vi "Generate Patch Sequence Images-retd.vi"(4 "Green":path[](array[path]), 5 "Red":path[](array[path]), 6 "Predominant ROI type":T1=enum."Comp. volume", 7 "Imaging Protocol":T2=enum."Live Imaging", 8 "error in (no error)":errorcluster, 9 "Green TIFF handles":i32[](array[numeric]), 10 "Red TIFF handles":i32[](array[numeric]), 11 "TDMS file path & name":path) -> (0 "error out":errorcluster, 2 "Destination fiolder":path)   [LabVIEW 2020]
uses:
  Typedefs/Imaging Protocols enum.ctl
  Typedefs/ROI ID Enum.ctl
  User Interface/Visualisation/Functional Imaging Viewer/SubVIs/Experiment header interface/Typedefs/Save-Load-Save as-Load last enum.ctl
  User Interface/Visualisation/Functional Imaging Viewer/SubVIs/Experiment header interface/Typedefs/Header file type enum.ctl
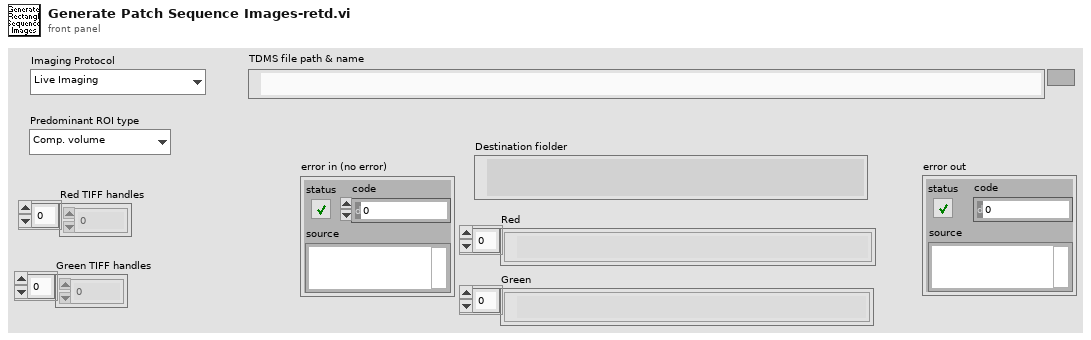
[diagram p1: front panel]
types:
  T1 = typedef "ROI ID Enum.ctl" = enum16{"Point", "MiniScan", "Comp. MiniScan", "Rectangle", "Comp. volume", "Arb. plane point", "None"}
  T2 = typedef "Imaging Protocols enum.ctl" = enum16{"AOL Z-Stack", "Motor Z Stack", "Functional Acquisition", "Single Plane Acquisition", "Volume Acquisition", "Live Imaging", "Live Plane Imaging", "Live Volume Imaging"}
  T3 = typedef "Header file type enum.ctl" = enum16{"All parameters", "Params for funct acq w ROI or mscn", "Params for funct acq w rectangles", "Live imaging header parameters", "AOL Parameters"}
  T4 = typedef "Header file type enum.ctl" = enum16{"All parameters", "Login", "Global Parameters", "Imaging Modes", "Time Series", "Motor Zstack", "AOL Zstack", "Functional Imaging", "Movement Correction", "Calibration Setup", "Statistics", "Biology Information"}
  T5 = typedef "Save-Load-Save as-Load last enum.ctl" = enum16{"Save file", "Save file as", "Load file", "Load last file"}
  T6 = typedef "Header parameters cluster-ALL-retd.ctl" = cluster{"Imaging Protocol":T2, "Number of POI":u16, "Number of Miniscans":u16, "Number of Trials":u16, "Number of Cycles ":u64, "# Averaged Frames":u16, "Laser power (%)":u8, "Pockels":dbl, "Acquisition Length (sec)":dbl, "Fill time (us)":dbl, "POI Dwell time (us)":dbl, "Miniscan Dwell time per pixel (us)":dbl, "PMT 1":dbl, "PMT 2":dbl, "Back Apperture":dbl, "Zoom":dbl, "Frame Size":T7, "Center Frequency":dbl, "Field of View":dbl, "DwellTime (us)":dbl, "Wavelength (nm)":dbl, "AOL Z":dbl, "AOL Mode":T8, "GridXY":dbl, "GridZ":dbl, "TriggerDelay (sec)":dbl, "Number of Pixels in Miniscan":u16, "Experiment folder path":path, "X centre":dbl, "Y centre":dbl, "Angle (degrees)":dbl, "Plane Mode":T9, "Software version":dbl, "Objective":T10, "MotorZ Calibration":u32, "Pockels Calibration":u32, "Threshold":u16[], "Video length (sec)":dbl, "Frame rate (fps)":u8, "Rectangle ROI length (pixels)":u16, "Rectangle ROI height (pixels)":u16}
  T7 = typedef "Frame Size.ctl" = u16
  T8 = typedef "AOL modes.ctl" = enum16{"Raster", "Structural", "Pointing", "Mini Scan", "Alignment"}
  T9 = typedef "Plane Mode.ctl" = u16
  T10 = typedef "Objective selector control enum.ctl" = string
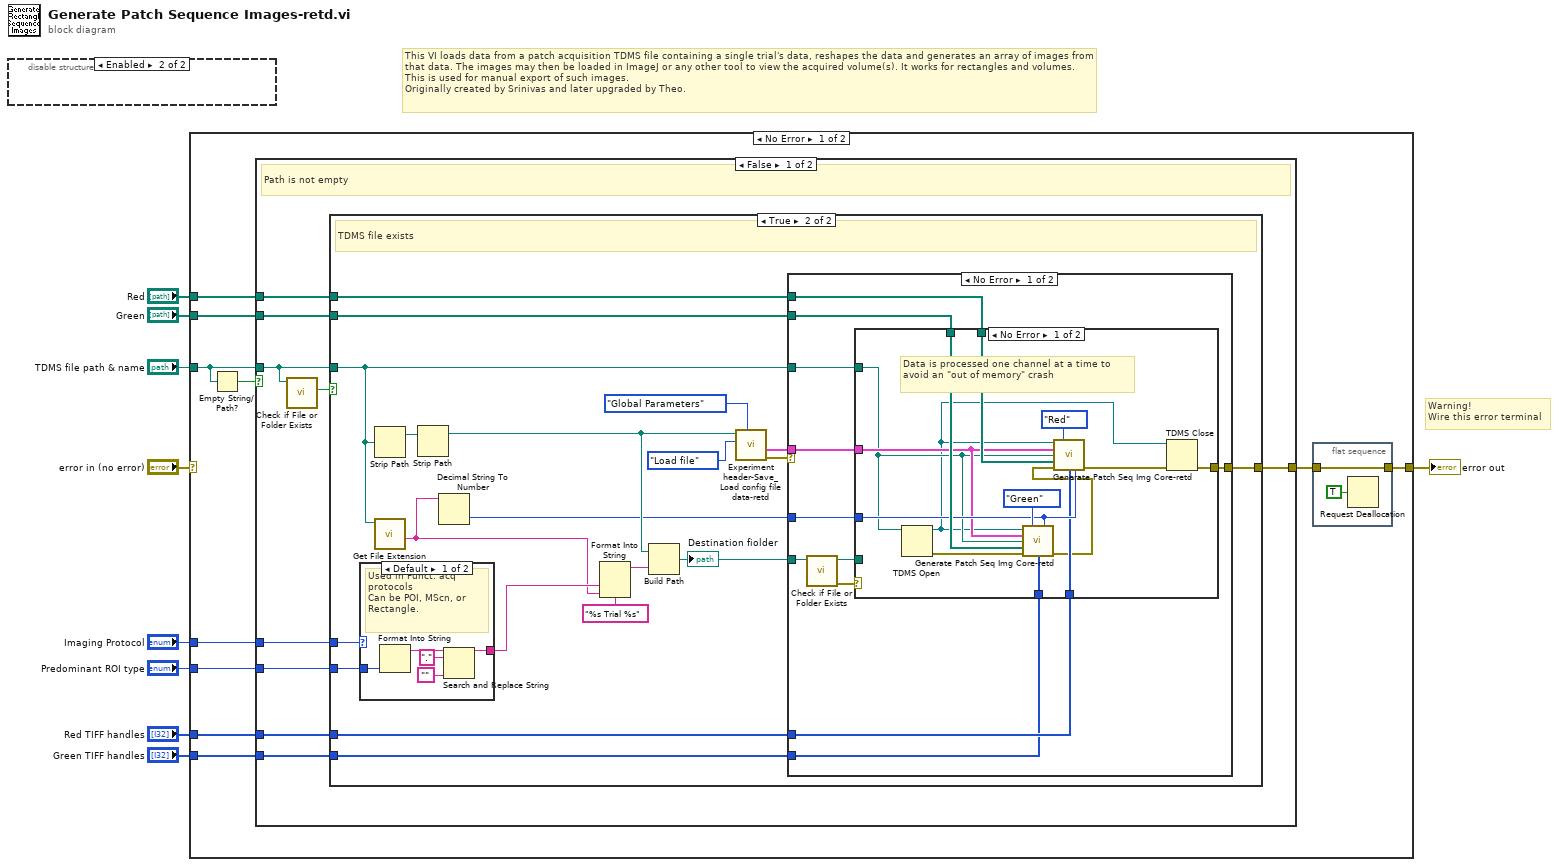
[diagram p0: block diagram]
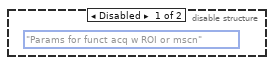
[diagram p2: hidden frame]
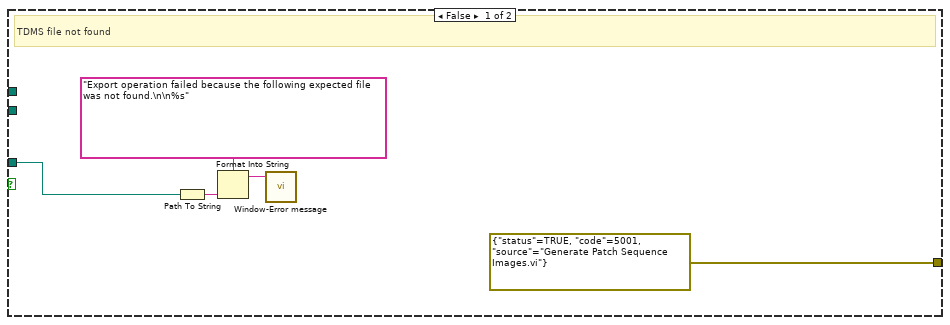
[diagram p3: hidden frame]
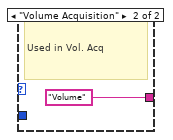
[diagram p6: hidden frame]
diagram:
  # "This VI loads data from a patch acquisition TDMS file containing a single trial's data, reshapes the data and generates an array of images from that data. The images may then be loaded in ImageJ or any other tool to view the acquired volume(s). It works for rectangles and volumes. This is used for manual export of such images.\nOriginally created by Srinivas and later upgraded by Theo."
  # "Warning!\nWire this error terminal"
  n1 = disable-structure shown="Enabled" {
    frame Disabled {
      (unwired) Header_file_type_enum."Params for funct acq w ROI or mscn" ("Header file type")
    }
    frame Enabled {
    }
  }
  n2 = case shown="No Error" "error in (no error)" {
    selector: "error in (no error)" -> [_ w88]
    tunnel: "TDMS file path & name" -> [w18 _]
    tunnel: "Imaging Protocol" -> [w17 _]
    tunnel: "Predominant ROI type" -> [w16 _]
    tunnel: "Green" -> [w14 _]
    tunnel: "Red" -> [w13 _]
    tunnel: "Red TIFF handles" -> [w12 _]
    tunnel: "Green TIFF handles" -> [w11 _]
    tunnel: [w10 w88] -> w2
    frame No Error {
      n3 = Empty String/Path?(string/path=w18) -> (empty?=w19:bool)
      n4 = case shown="False" w19 {
        tunnel: w18 -> [w29 _]
        tunnel: [w28 _] -> w15
        tunnel: w17 -> [w27 _]
        tunnel: w16 -> [w26 _]
        tunnel: w14 -> [w25 _]
        tunnel: w13 -> [w24 _]
        tunnel: w12 -> [w23 _]
        tunnel: w11 -> [w22 _]
        frame False {
          # "Path is not empty"
          n5 = call <vilib>:"Check if File or Folder Exists.vi"("path"=w29) -> ("file or folder exists?"=w30:bool)  [unwired: 8 in, 2 out]
          n6 = case shown="True" w30 {
            tunnel: w29 -> [w34 w55]
            tunnel: [errorcluster {"status"=TRUE, "code"=5001, "source"="Generate Patch Sequence Images.vi"} ("error IO") w53] -> w28
            tunnel: w27 -> [_ w51]
            tunnel: w26 -> [_ w50]
            tunnel: w25 -> [_ w49]
            tunnel: w24 -> [_ w48]
            tunnel: w23 -> [_ w39]
            tunnel: w22 -> [_ w38]
            frame False {
              # "TDMS file not found"
              n7 = Path To String(path=w34) -> (string=w33:string)
              n8 = Format Into String(format string="Export operation failed because the following expected file was not found.\n\n%s", w33) -> (resulting string=w32:string)  [unwired: 2 in, 1 out]
              n9 = call "Window-Error message.vi"("Message"=w32) -> ()  [unwired: 10 in, 1 out]
            }
            frame True {
              # "TDMS file exists"
              n10 = case shown="Default" w51 {
                tunnel: w50 -> [w86 _]
                tunnel: [w82 "Volume" ("result string")] -> w44
                frame Default {
                  # "Used in Funct. acq protocols\nCan be POI, MScn, or Rectangle."
                  n11 = Format Into String(w86) -> (resulting string=w85:string)  [unwired: 3 in, 1 out]
                  n12 = Search and Replace String(input string=w85, search string=".", replace string="" ("replace string (\"\")")) -> (result string=w82:string)  [unwired: 5 in, 3 out]
                }
                frame "Volume Acquisition" {
                  # "Used in Vol. Acq"
                }
              }
              n13 = Strip Path(path=w55) -> (stripped path=w46:path)  [unwired: 1 out]
              n14 = call <vilib>:"Get File Extension.vi"("file"=w55) -> ("filename without extension"=w42:string)  [unwired: 6 in, 4 out]
              n15 = Strip Path(path=w46) -> (stripped path=w54:path)  [unwired: 1 out]
              n16 = Decimal String To Number(string=w42) -> (number=w47:i32)  [unwired: 2 in, 1 out]
              n17 = Format Into String(format string="%s Trial %s", w44, w42) -> (resulting string=w43:string)  [unwired: 2 in, 1 out]
              n18 = Build Path(base path=w54, name or relative path=w43) -> (appended path=w52:path)
              "Destination fiolder" <- w52
              n19 = call "Experiment header-Save_Load config file data-retd.vi"("Header file type"=Header_file_type_enum."Global Parameters", "Function"=Save-Load-Save_as-Load_last_enum."Load file", "Experiment data folder path"=w54) -> ("error out"=w40:errorcluster, "All header parameters out"=w41:T6)  [unwired: 7 in]
              n20 = case shown="No Error" w40 {
                tunnel: w52 -> [w66 _]
                tunnel: w55 -> [w65 _]
                tunnel: w41 -> [w63 _]
                tunnel: [w64 _] -> w53
                tunnel: w49 -> [w62 _]
                tunnel: w48 -> [w61 _]
                tunnel: w47 -> [w60 _]
                tunnel: w39 -> [w57 _]
                tunnel: w38 -> [w56 _]
                frame No Error {
                  n21 = call <vilib>:"Check if File or Folder Exists.vi"("path"=w66) -> ("error out"=w58:errorcluster, "dup path"=w59:path)  [unwired: 8 in, 1 out]
                  n22 = case shown="No Error" w58 {
                    selector: w58 -> [_ w81]
                    tunnel: w59 -> [_ _]
                    tunnel: w65 -> [w71 _]
                    tunnel: w63 -> [w72 _]
                    tunnel: [w76 w81] -> w64
                    tunnel: w62 -> [w79 _]
                    tunnel: w61 -> [w78 _]
                    tunnel: w60 -> [w77 _]
                    tunnel: w57 -> [w75 _]
                    tunnel: w56 -> [w74 _]
                    frame No Error {
                      # "Data is processed one channel at a time to avoid an \"out of memory\" crash"
                      n23 = TDMS Open(11:w71) -> (0:w70:errorcluster, 3:w69:refnum<k34>)  [unwired: 6 in]
                      n24 = call "Generate Patch Seq Img Core-retd.vi"("tdms file ref"=w69, "Channel to process"=enum16{"Red", "Green"}."Green", "All header parameters"=w72, "TDMS file path & name"=w71, "Patch Image Folder"=w79, "error in (no error)"=w70, "TIFF file handles"=w74, "Trial Number"=w77) -> ("error out"=w68:errorcluster)  [unwired: 6 in, 1 out]
                      n25 = call "Generate Patch Seq Img Core-retd.vi"("tdms file ref"=w69, "Channel to process"=enum16{"Red", "Green"}."Red", "All header parameters"=w72, "TDMS file path & name"=w71, "Patch Image Folder"=w78, "error in (no error)"=w68, "TIFF file handles"=w75, "Trial Number"=w77) -> ("error out"=w67:errorcluster)  [unwired: 6 in, 1 out]
                      n26 = TDMS Close(8:w67, 11:w69) -> (0:w76:errorcluster)  [unwired: 1 out]
                    }
                    frame Error {
                    }
                  }
                }
                frame Error {
                  # "Error reporting handled inside the subVI."
                }
              }
            }
          }
        }
        frame True {
          # "Path is empty"
        }
      }
      n27 = flat-sequence {
        tunnel: w15 -> [w20]
        tunnel: [w20] -> w10
        frame #0 {
          n28 = Request Deallocation(TRUE ("flag")) -> ()
        }
      }
    }
    frame Error {
    }
  }
  "error out" <- w2
